vi "Msg To Nested.vi"(8 "Alias":string, 9 "Priority?":bool, 10 "Msg":refnum<class "Msg.lvclass">, 11 "jettl Queue Actor in":refnum<class "jettl Queue Actor.lvclass">) -> (0 "error out":errorcluster)   [LabVIEW 2021, in "jettl.lvlib" / "jettl Queue Actor.lvlib" / "jettl Queue Actor.lvclass"]
uses:
  jettl Queue Actor.lvclass
  Actor/Msg/Msg.lvclass
  jettl Queue Actor.lvclass/jettl Queue Actor.ctl
  jettl.lvlib
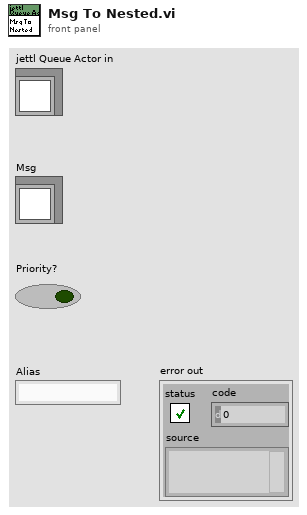
[diagram p1: front panel]
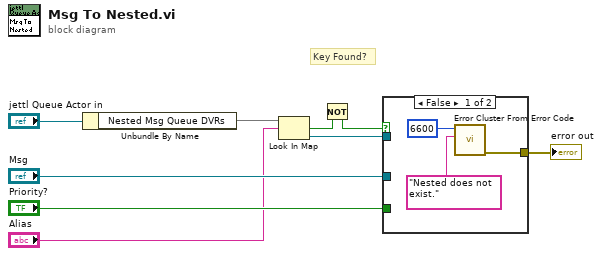
[diagram p0: block diagram]
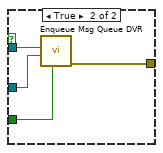
[diagram p2: hidden frame]
diagram:
  # "Key Found?"
  n1 = Unbundle By Name("jettl Queue Actor in") -> ("Nested Msg Queue DVRs"=w5:map{string, refnum<data-value>})
  n2 = Look In Map(map=w5, key="Alias") -> (key not found?=w2:bool, value=w3:refnum<data-value>)  [unwired: 1 in]
  n3 = Not(x=w2) -> (.not. x?=w1:bool)
  n4 = case shown="False" w1 {
    tunnel: [w12 w16] -> w9
    tunnel: "Msg" -> [_ w15]
    tunnel: "Priority?" -> [_ w14]
    tunnel: w3 -> [_ w13]
    frame False {
      n5 = call <vilib>:"Error Cluster From Error Code.vi"("error message (\"\")"="Nested does not exist." ("error message (\"\")"), "error code (0)"=6600) -> ("error out"=w12:errorcluster)  [unwired: 7 in]
    }
    frame True {
      n6 = call "Enqueue Msg Queue DVR.vi"("Priority?"=w14, "Msg"=w15, "Msg Queue DVR"=w13) -> ("error out"=w16:errorcluster)  [unwired: 8 in]
    }
  }
  "error out" <- w9
